vi "Write TempData.vi"(8 "error in (no error)":errorcluster, 10 "TempData":cluster{"Temp":dbl, "Humid":dbl}, 11 "SetTemp Message":refnum<class "SetTemp Message.lvclass">) -> (0 "error out":errorcluster, 3 "SetTemp Message":refnum<class "SetTemp Message.lvclass">)   [LabVIEW 2018, in "QMH_Class.lvlib" / "TestManager.lvlib" / "SetTemp Message.lvclass"]
uses:
  SetTemp Message.lvclass
  SetTemp Message.lvclass/SetTemp Message.ctl
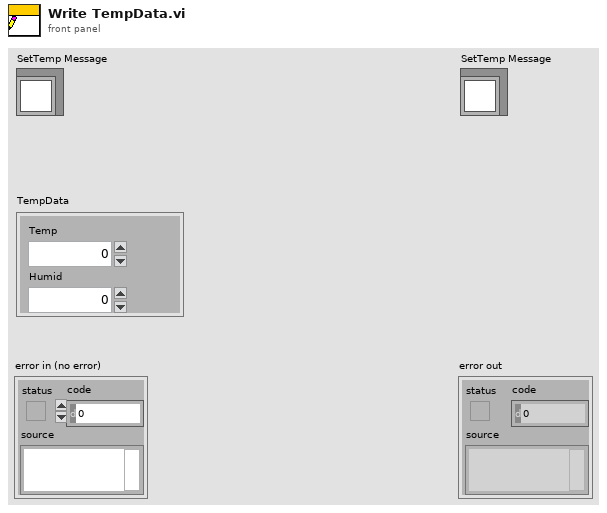
[diagram p1: front panel]
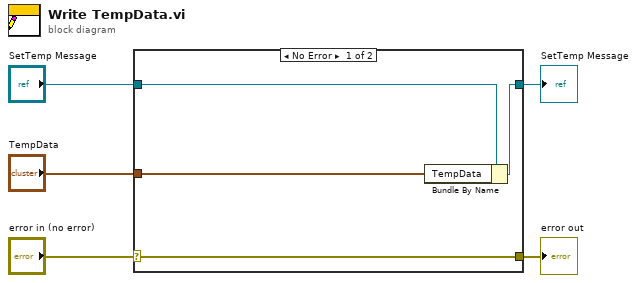
[diagram p0: block diagram]
diagram:
  n1 = case shown="No Error" "error in (no error)" {
    selector: "error in (no error)" -> [w9 w10]
    tunnel: [w9 w10] -> w4
    tunnel: [w7 w11] -> w2
    tunnel: "SetTemp Message" -> [w8 w11]
    tunnel: "TempData" -> [w6 _]
    frame No Error {
      n2 = Bundle By Name(cluster=w8, "TempData"=w6) -> (w7:refnum<class "SetTemp Message.lvclass">)
    }
    frame Error {
    }
  }
  "error out" <- w4
  "SetTemp Message" <- w2
